vi "Read Data.vi"(8 "Error In":errorcluster, 11 "Writer In":refnum<class "Writer.lvclass">) -> (0 "Error Out":errorcluster, 2 "Value":u8[](array[numeric]), 3 "Writer Out":refnum<class "Writer.lvclass">)   [LabVIEW 2018, in "Toolkit.lvlib" / "Writer.lvclass"]
doc: "Gets the current MessagePack data from the internal encoder's buffer."
uses:
  Writer.lvclass
  Writer.lvclass/Writer.ctl
  Status/Read Is Error.vi
  Status/Read Status.vi
  Status/Read Status Message.vi
  Utility/Status Code.vi
  <vilib>/Utility/error.llb/Error Cluster From Error Code.vi
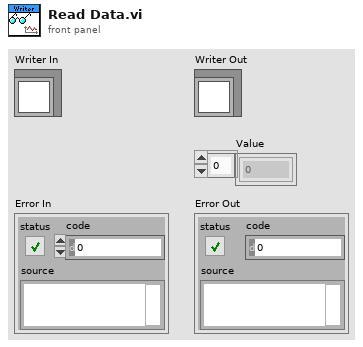
[diagram p1: front panel]
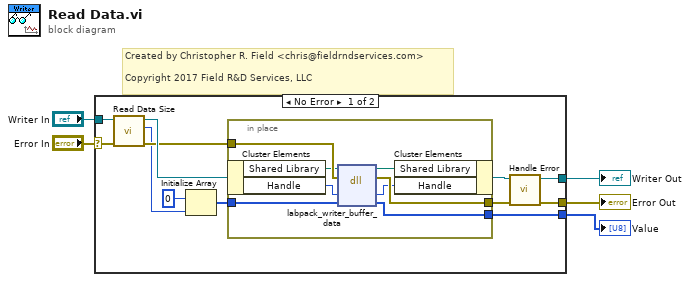
[diagram p0: block diagram]
diagram:
  # "Created by Christopher R. Field <chris@fieldrndservices.com>\n\nCopyright 2017 Field R&D Services, LLC"
  n1 = case shown="No Error" "Error In" {
    selector: "Error In" -> [w15 w26]
    tunnel: "Writer In" -> [w16 w27]
    tunnel: [w10 w27] -> w3
    tunnel: [w8 w26] -> w2
    tunnel: [w6 _] -> w1
    frame No Error {
      n2 = call "Read Data Size.vi"("Error In"=w15, "Writer In"=w16) -> ("Error Out"=w13:errorcluster, "Count"=w11:u64, "Writer Out"=w14:refnum<class "Writer.lvclass">)  [unwired: 7 in]
      n3 = Initialize Array(u8 0, w11) -> (w7:u8[])
      n4 = in-place {
        in-place-border: w13 -> [w25]
        in-place-border: [w24] -> w9
        in-place-border: w7 -> [w19]
        in-place-border: [w18] -> w6
        n5 = in-place-cluster #1(w14) -> ("Shared Library"=w21:path, "Handle"=w23:u64)
        n6 = dll-call lib="D:/Users/cfield/Code/MessagePack/LabPack/LabVIEW/trunk/src/LabPack/Private/labpack-x64.dll" fn="labpack_writer_buffer_data"(path in=w21, error in=w25, "writer"=w23, "buffer"=w19) -> (path out=w20:path, error out=w24:errorcluster, "writer"=w22:u64, "buffer"=w18:u8[])  [unwired: 2 in]
        n7 = in-place-cluster #1("Shared Library"=w20, "Handle"=w22) -> (w17:refnum<class "Writer.lvclass">)
      }
      n8 = call "Handle Error.vi"("Error In"=w9, "Writer In"=w17) -> ("Error Out"=w8:errorcluster, "Writer Out"=w10:refnum<class "Writer.lvclass">)  [unwired: 8 in]
    }
    frame Error {
    }
  }
  "Writer Out" <- w3
  "Error Out" <- w2
  "Value" <- w1
